vi "Set Serial Settings.vi"(8 "error in (no error)":errorcluster, 11 "Quartz in":refnum<class "Quartz.lvclass">) -> (0 "error out":errorcluster, 3 "Quartz out":refnum<class "Quartz.lvclass">)   [LabVIEW 2016, in "Quartz.lvclass"]
uses:
  Quartz.lvclass
  Desktop/platinum-modbus-driver/omega_engineering-platinum-modbus-driver-671bd10261c3/Labview Source Code/Platinum Serial Modbus/Platinum_MB_SerHandle.ctl
  Desktop/platinum-modbus-driver/omega_engineering-platinum-modbus-driver-671bd10261c3/Labview Source Code/Platinum Serial Modbus/Platinum_MB_serMode.ctl
  Desktop/platinum-modbus-driver/omega_engineering-platinum-modbus-driver-671bd10261c3/Labview Source Code/Platinum Serial Modbus/Platinum_MB_serFlowControl.ctl
  Desktop/platinum-modbus-driver/omega_engineering-platinum-modbus-driver-671bd10261c3/Labview Source Code/Platinum Serial Modbus/Platinum_MB_serParity.ctl
  Quartz.lvclass/Quartz.ctl
  LightBox/LightBox.lvclass
  <vilib>/Utility/config.llb/NI_LVConfig.lvlib
  <vilib>/Utility/config.llb/Read Key (String).vi
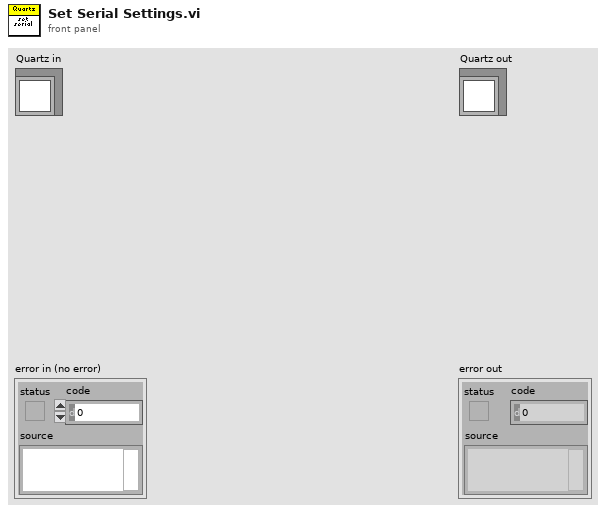
[diagram p1: front panel]
types:
  T1 = typedef "Platinum_MB_serFlowControl.ctl" = enum16{"None", "XON_XOFF", "RTS_CTS", "XON_XOFF_and_RTS_CTS", "DTR_DSR", "XON_XOFF_and_DTR_DSR"}
  T2 = typedef "Platinum_MB_serMode.ctl" = enum16{"RTU", "ASCII"}
  T3 = typedef "Platinum_MB_serParity.ctl" = enum16{"None", "Odd", "Even", "Mark", "Space"}
  T4 = typedef "Platinum_MB_SerHandle.ctl" = cluster{"VISAResourceName":string, "Mode":T2, "Timeout":u32, "FlowControl":T1, "Parity":T3, "BaudRate":u32, "SlaveAddress":u8}
  T5 = typedef "NI_LVConfig.lvlib/Config Data RefNum.ctl" = refnum<k1>
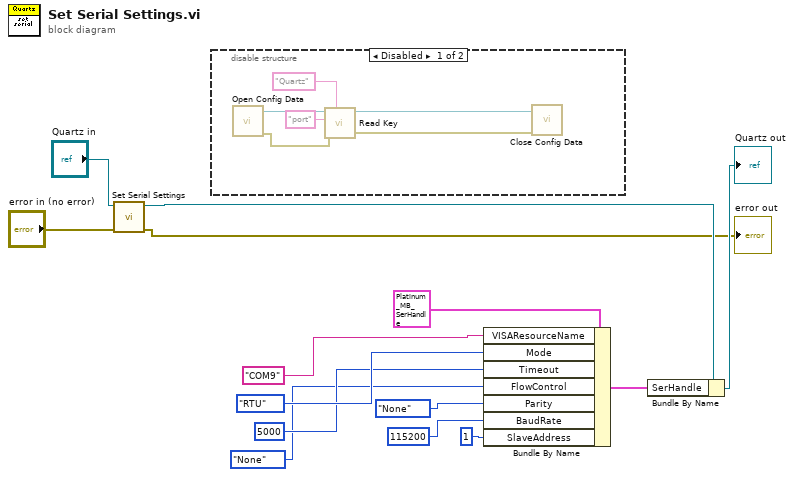
[diagram p0: block diagram]
diagram:
  n1 = call-parent "Set Serial Settings.vi"("error in (no error)"="error in (no error)", "LightBox in"="Quartz in") -> ("error out"=→"error out":errorcluster, "LightBox out"=w5:refnum<class "Quartz.lvclass">)  [unwired: 8 in]
  n2 = disable-structure shown="Disabled" {
    frame Disabled {
      n3 = call <vilib>:"Open Config Data.vi"() -> ("error out"=w17:errorcluster, "refnum"=w20:T5)  [unwired: 9 in, 1 out]
      n4 = call-poly <vilib>:"Read Key.vi"("section"="Quartz", "error in (no error)"=w17, "key"="port", "refnum"=w20) -> ("error out"=w15:errorcluster, "refnum out"=w16:T5)  [unwired: 4 in, 2 out]
      n5 = call <vilib>:"Close Config Data.vi"("error in (no error)"=w15, "refnum"=w16) -> ()  [unwired: 8 in, 2 out]
    }
    frame Enabled {
    }
  }
  n6 = Bundle By Name(cluster=T4 {"VISAResourceName"="COM9", "Mode"=enum."RTU", "Timeout"=500, "FlowControl"=enum."None", "Parity"=enum."None", "BaudRate"=9600, "SlaveAddress"=1} ("SerHandle"), "VISAResourceName"="COM9", "Mode"=Platinum_MB_serMode."RTU", "Timeout"=u32 5000, "FlowControl"=Platinum_MB_serFlowControl."None", "Parity"=Platinum_MB_serParity."None", "BaudRate"=u32 115200, "SlaveAddress"=u8 1) -> (w12:T4)
  n7 = Bundle By Name(cluster=w5, "SerHandle"=w12) -> (→"Quartz out":refnum<class "Quartz.lvclass">)
